vi "Time Counter.vi"(9 "Action":enum16{"Start", "Stop"}(ring)) -> (1 "Elapsed":u32)   [LabVIEW 2015]
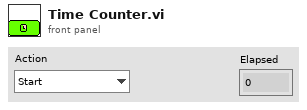
[diagram p1: front panel]
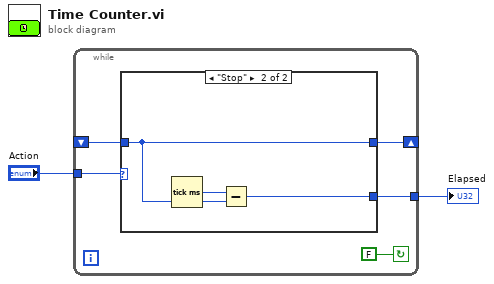
[diagram p0: block diagram]
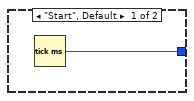
[diagram p2: hidden frame]
diagram:
  n1 = while {
    tunnel: "Action" -> [w6]
    shift-right: [w5] -> _
    shift-left: _ -> [w4]
    tunnel: [w3] -> w1
    stop <- FALSE continue-if-true
    n2 = case shown="\"Stop\"" w6 {
      tunnel: [w8 w9] -> w5
      tunnel: w4 -> [_ w9]
      tunnel: [_ w10] -> w3
      frame "Start", Default {
        n3 = Tick Count (ms)() -> (millisecond timer value=w8:u32)
      }
      frame "Stop" {
        n4 = Tick Count (ms)() -> (millisecond timer value=w11:u32)
        n5 = Subtract(x=w11, y=w9) -> (x-y=w10:u32)
      }
    }
  }
  "Elapsed" <- w1
